vi "SetInstrumentFromMarker.vi"(8 "error in (no error)":errorcluster, 11 "SpecAnBase in":refnum<class "SpecAnBase.lvclass">) -> (0 "error out":errorcluster, 3 "SpecAnBase out":refnum<class "SpecAnBase.lvclass">)   [LabVIEW 2018, in "SpecAnPlugins.lvlib" / "SpecAnBase.lvclass"]
doc: "This VI makes the Active Marker frequency to be the start frequency, the stop frequency, or the center frequency. It can also make the active marker amplitude to be the reference level. This affects either the Frequency Start, Frequency Stop, or the Reference Level property. \n\nNotes:\n\n(1) This VI INVALIDATES the Frequency Start and Frequency Stop property values or INVALIDATES Reference Level property.\n\n(2) This VI will return error Marker Not Enabled if the active marker is not enabled."
uses:
  SpecAnBase.lvclass
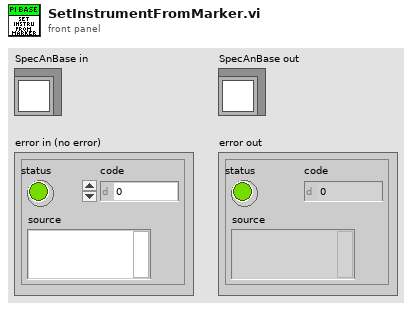
[diagram p1: front panel]
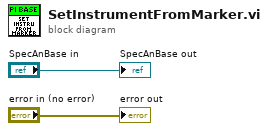
[diagram p0: block diagram]
diagram:
  "error out" <- "error in (no error)"
  "SpecAnBase out" <- "SpecAnBase in"
